vi "SerialServer.vi"(5 "Stop Refnum":refnum<vi>, 6 "Local Port":u16=16505, 7 "FPGA VI Reference In":refnum<k20>) -> (3 "FPGA VI Reference Out":refnum<k20>)   [LabVIEW 2012]
panel:
  out "error out":errorcluster
  out "OverRunError":bool
  in  "Flush on close":bool
  out "UART TX count":u64
  out "UART RX count":u64
  out "TCP Bytes Out":u64
  out "Elements in UART TX Queue":i32
  out "Elements in UART RX Queue":i32
  out "TCP Bytes In":u64
  out "connection ID":refnum<k5>
  out "Connected?":bool
  out "Stopped?":bool caption="BeenStopped?"
  out "remote address":string
  out "Remote Port":u16
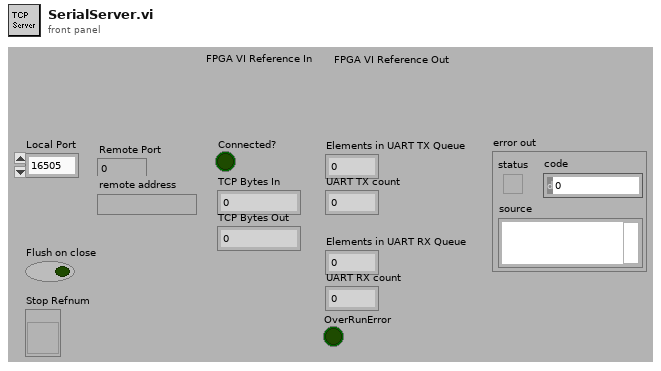
[diagram p1: front panel]
types:
  T1 = enum16{"Standard", "Buffered", "CRLF", "Immediate"}
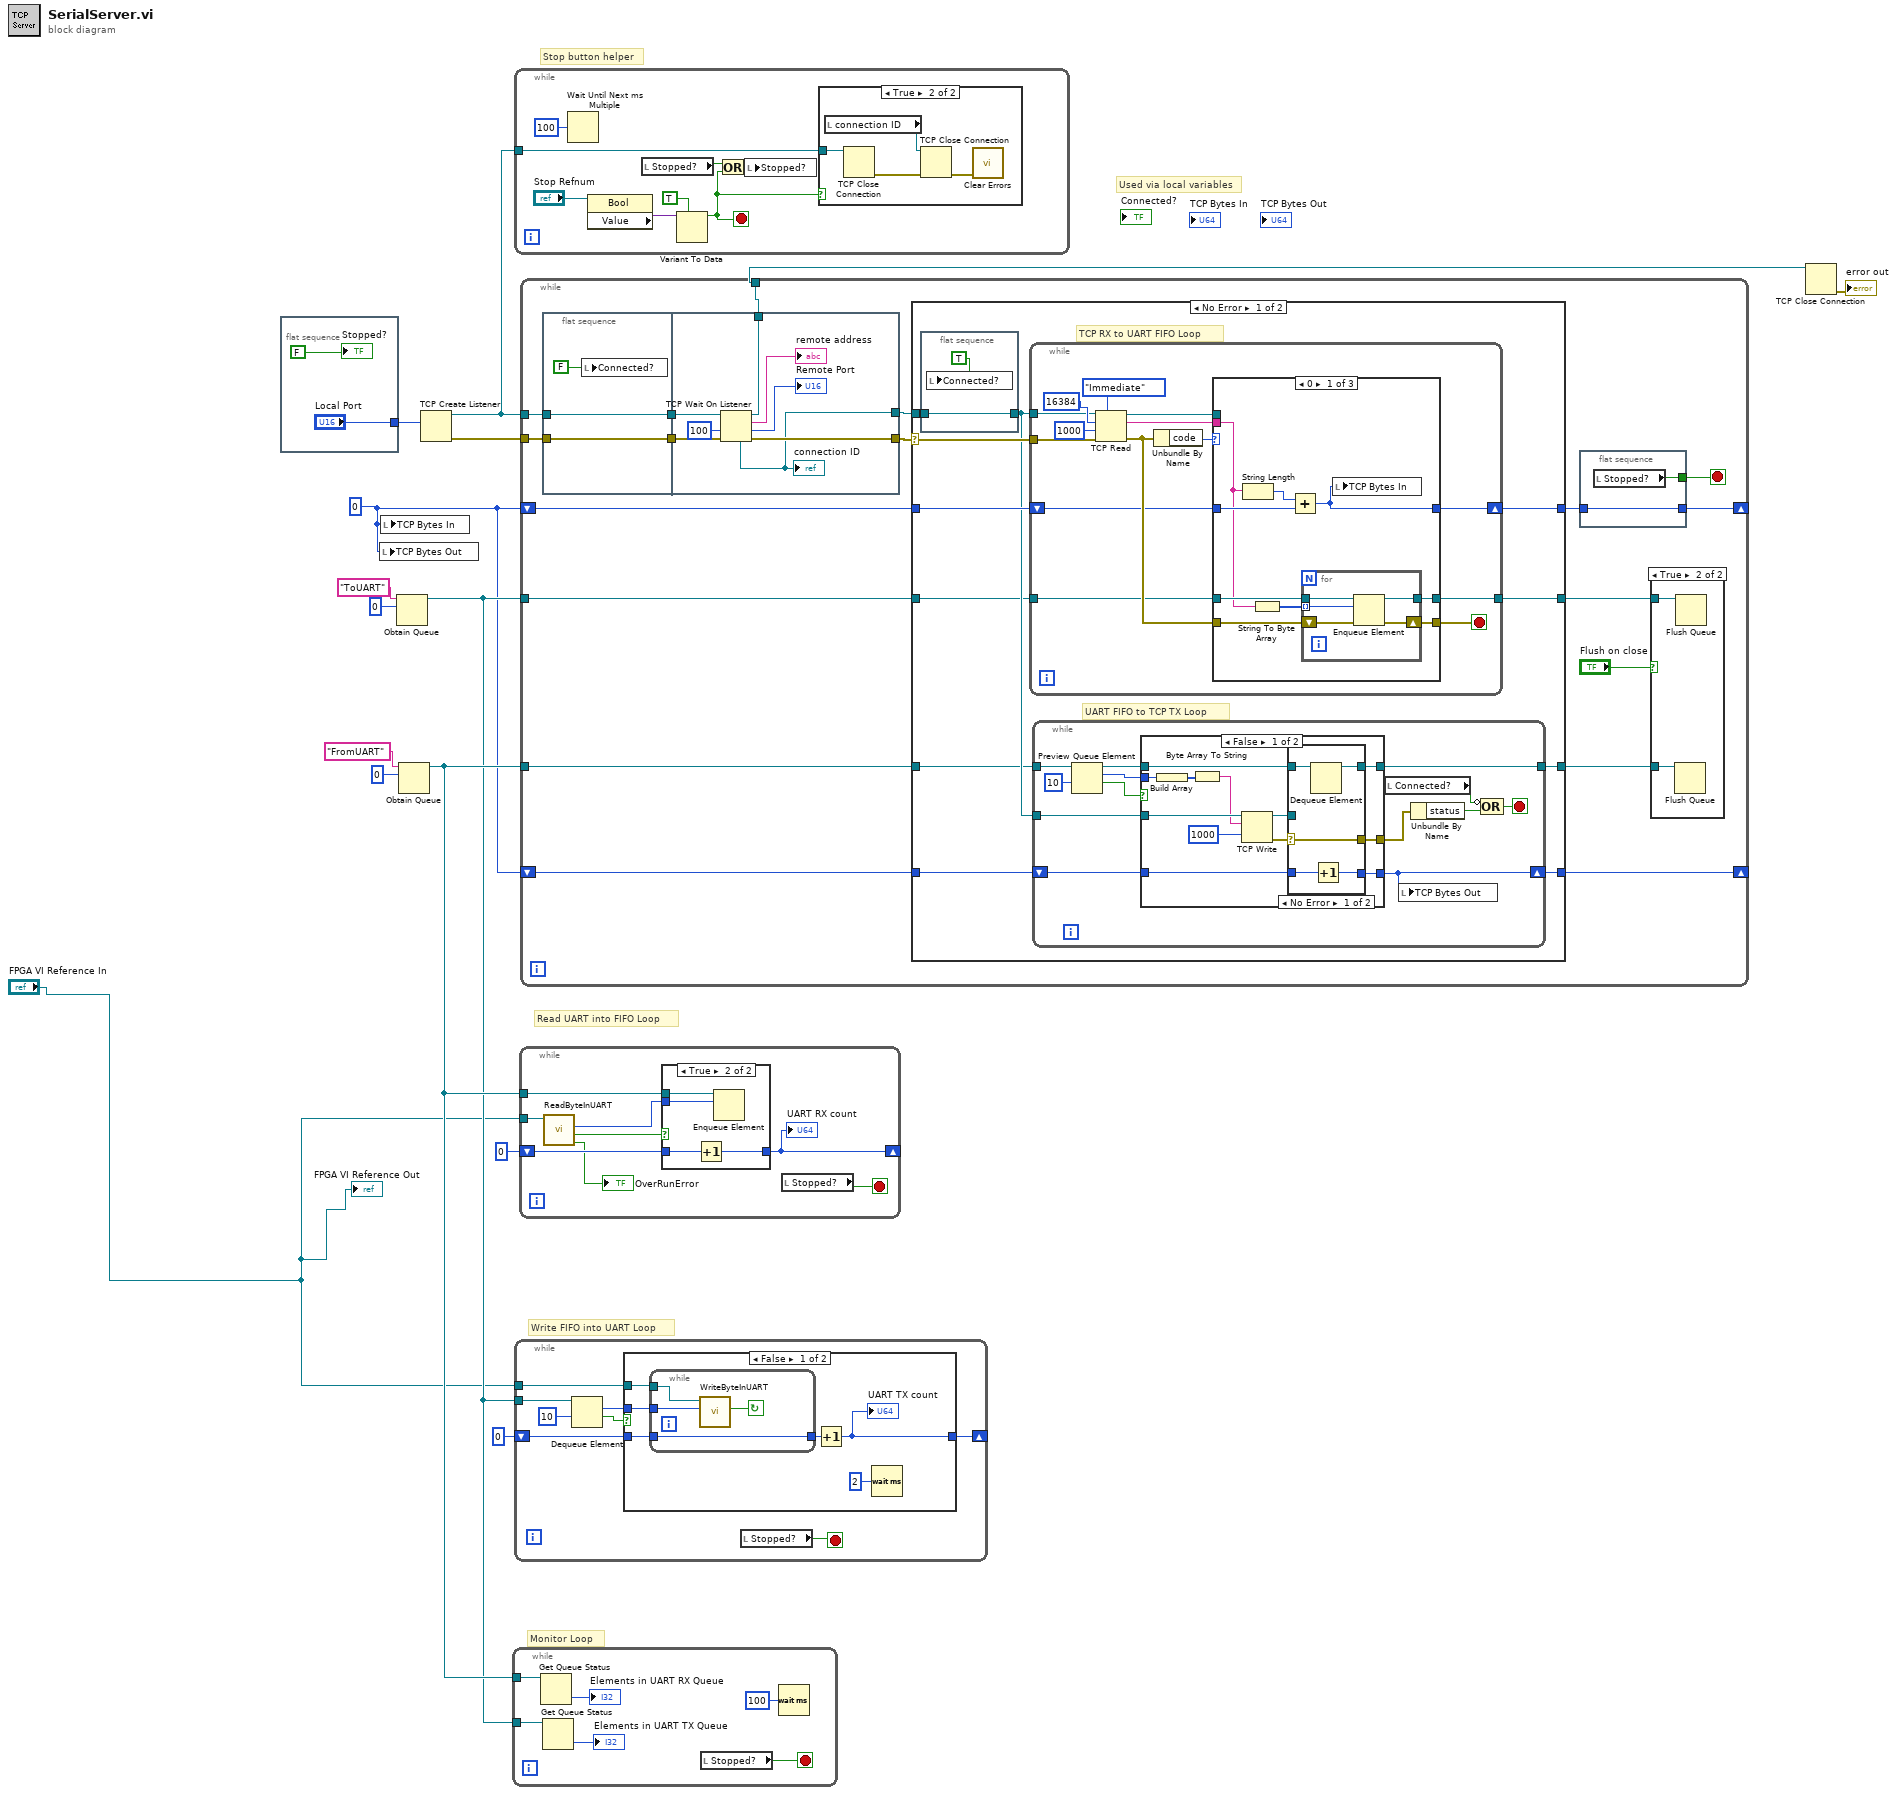
[diagram p0: block diagram]
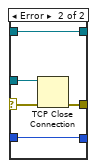
[diagram p6: hidden frame]
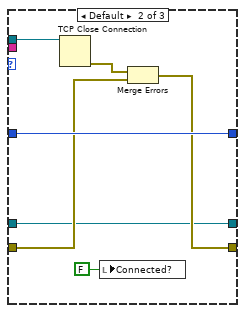
[diagram p8: hidden frame]
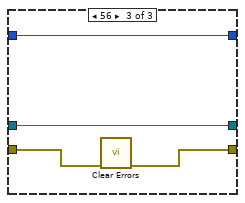
[diagram p9: hidden frame]
diagram:
  w7 = u64 0
  # "Monitor Loop"
  # "Write FIFO into UART Loop"
  # "Read UART into FIFO Loop"
  # "Stop button helper"
  # "Used via local variables"
  n1 = flat-sequence {
    tunnel: ["Local Port"] -> w2
    frame #0 {
      "Stopped?" <- FALSE ("Stopped?")
    }
  }
  n2 = local write "TCP Bytes Out"(w7) -> ()
  n3 = local write "TCP Bytes In"(w7) -> ()
  n4 = Obtain Queue(name (unnamed)="ToUART", element data type=u8 0) -> (queue out=w8:refnum<queue>)  [unwired: 3 in, 2 out]
  n5 = Obtain Queue(name (unnamed)="FromUART", element data type=u8 0) -> (queue out=w9:refnum<queue>)  [unwired: 3 in, 2 out]
  n6 = TCP Create Listener(10:w2) -> (0:w15:errorcluster, 3:w14:refnum<k5>)  [unwired: 1 in, 4 out]
  n7 = while {
    tunnel: w9 -> [w21]
    tunnel: w8 -> [w19]
    stop <- w23 stop-if-true
    n8 = Get Queue Status(queue=w21) -> (# elements in queue=→"Elements in UART RX Queue":i32)  [unwired: 1 in, 8 out]
    n9 = Get Queue Status(queue=w19) -> (# elements in queue=→"Elements in UART TX Queue":i32)  [unwired: 1 in, 8 out]
    n10 = local read "Stopped?"() -> (w23:bool)
    n11 = Wait (ms)(milliseconds to wait=u32 100) -> ()  [unwired: 1 out]
  }
  n12 = while {
    tunnel: w14 -> [w30]
    stop <- w24 stop-if-true
    n13 = Wait Until Next ms Multiple(millisecond multiple=u32 100) -> ()  [unwired: 1 out]
    n14 = property class="Bool"(reference="Stop Refnum") -> ("Value"=w29:variant)  [unwired: 1 in, 2 out]
    n15 = local read "Stopped?"() -> (w25:bool)
    n16 = Variant To Data(type=TRUE ("stop"), Variant=w29) -> (data=w24:bool)  [unwired: 1 in, 1 out]
    n17 = Or(x=w25, y=w24) -> (x .or. y?=w26:bool)
    n18 = local write "Stopped?"(w26) -> ()
    n19 = case shown="True" w24 {
      tunnel: w30 -> [_ w32]
      frame False {
      }
      frame True {
        n20 = local read "connection ID"() -> (w34:refnum<k5>)
        n21 = TCP Close Connection(connection ID=w32) -> (error out=w33:errorcluster)  [unwired: 1 in, 2 out]
        n22 = TCP Close Connection(connection ID=w34, error in (no error)=w33) -> (error out=w35:errorcluster)  [unwired: 2 out]
        n23 = call <vilib>:"Clear Errors.vi"("error in (no error)"=w35) -> ()  [unwired: 7 out]
      }
    }
  }
  n24 = while {
    tunnel: w8 -> [w43]
    shift-right: [w37] -> _
    shift-left: u64 0 -> [w38]
    tunnel: "FPGA VI Reference In" -> [w36]
    stop <- w39 stop-if-true
    n25 = Dequeue Element(queue=w43, timeout in ms (-1)=10) -> (element=w40:u8, timed out?=w41:bool)  [unwired: 1 in, 2 out]
    n26 = case shown="False" w41 {
      tunnel: w40 -> [w49 _]
      tunnel: w38 -> [w48 w54]
      tunnel: [w46 w54] -> w37
      tunnel: w36 -> [w44 _]
      frame False {
        n27 = while {
          tunnel: w49 -> [w52]
          tunnel: w48 -> [w53]
          tunnel: [w53] -> w47
          tunnel: w44 -> [w50]
          stop <- w51 continue-if-true
          n28 = call "WriteByteInUART.vi"("Byte Value"=w52, "FPGA VI Reference In"=w50) -> ("Overflow?"=w51:bool)  [unwired: 2 in, 6 out]
        }
        n29 = Increment(x=w47) -> (x+1=w46:u64)
        "UART TX count" <- w46
        n30 = Wait (ms)(milliseconds to wait=u32 2) -> ()  [unwired: 1 out]
      }
      frame True {
      }
    }
    n31 = local read "Stopped?"() -> (w39:bool)
  }
  n32 = while {
    tunnel: w9 -> [w61]
    shift-right: [w59] -> _
    shift-left: u64 0 -> [w60]
    tunnel: "FPGA VI Reference In" -> [w58]
    stop <- w62 stop-if-true
    n33 = call "ReadByteInUART.vi"("FPGA VI Reference In"=w58) -> ("OverRunError"=→"OverRunError":bool, "Did Read Byte"=w55:bool, "Byte Value"=w57:u8)  [unwired: 8 out]
    n34 = case shown="True" w55 {
      tunnel: w61 -> [_ w67]
      tunnel: w57 -> [_ w66]
      tunnel: [w63 w65] -> w59
      tunnel: w60 -> [w63 w64]
      frame False {
      }
      frame True {
        n35 = Increment(x=w64) -> (x+1=w65:u64)
        n36 = Enqueue Element(queue=w67, element=w66) -> ()  [unwired: 1 in, 4 out]
      }
    }
    "UART RX count" <- w59
    n37 = local read "Stopped?"() -> (w62:bool)
  }
  n38 = while {
    tunnel: w14 -> [w84]
    tunnel: w15 -> [w85]
    shift-right: [w78] -> _
    shift-left: w7 -> [w80]
    tunnel: w8 -> [w77]
    tunnel: w9 -> [w74]
    shift-right: [w72] -> _
    shift-left: w7 -> [w73]
    tunnel: [w68] -> w4
    stop <- w81 stop-if-true
    n39 = flat-sequence {
      tunnel: w84 -> [w89]
      tunnel: w85 -> [w90]
      tunnel: [w90] -> w76
      tunnel: [w89] -> w75
      tunnel: w76 -> [w96]
      tunnel: w75 -> [w95]
      tunnel: [w94] -> w83
      tunnel: [w91] -> w82
      tunnel: [w92] -> w68
      frame #0 {
        n40 = local write "Connected?"(FALSE ("Connected?")) -> ()
      }
      frame #1 {
        n41 = TCP Wait On Listener(8:w96, 9:100 ("timeout ms (wait forever: -1)"), 11:w95) -> (0:w94:errorcluster, 1:→"Remote Port":u16, 2:→"remote address":string, 3:w92:refnum<k5>, 4:w91:refnum<k5>)  [unwired: 1 in]
        "connection ID" <- w91
      }
    }
    n42 = case shown="No Error" w83 {
      selector: w83 -> [w109 _]
      tunnel: w82 -> [w108 _]
      tunnel: w80 -> [w111 w193]
      tunnel: [w110 w193] -> w79
      tunnel: w77 -> [w103 w190]
      tunnel: w74 -> [w104 w191]
      tunnel: w73 -> [w106 w192]
      tunnel: [w105 w192] -> w72
      tunnel: [w102 w190] -> w71
      tunnel: [w101 w191] -> w70
      frame No Error {
        # "UART FIFO to TCP TX Loop"
        # "TCP RX to UART FIFO Loop"
        n43 = flat-sequence {
          tunnel: w108 -> [w149]
          tunnel: [w149] -> w107
          frame #0 {
            n44 = local write "Connected?"(TRUE ("Connected?")) -> ()
          }
        }
        n45 = while {
          tunnel: w109 -> [w157]
          shift-right: [w154] -> w110
          shift-left: w111 -> [w155]
          tunnel: w103 -> [w153]
          tunnel: w107 -> [w152]
          tunnel: [w151] -> w102
          stop <- w158 stop-if-true
          n46 = TCP Read(connection ID=w152, bytes to read=16384, error in (no error)=w157, 7:T1."Immediate" ("mode (standard)"), 9:1000 ("timeout ms (25000)")) -> (connection ID out=w160:refnum<k5>, data out=w159:string, error out=w161:errorcluster)
          n47 = Unbundle By Name(w161) -> ("code"=w162:i32)
          n48 = case shown="0" w162 {
            tunnel: w161 -> [w167 w183 w189]
            tunnel: w160 -> [_ w184 _]
            tunnel: w159 -> [w169 _ _]
            tunnel: [w166 w181 w188] -> w158
            tunnel: w155 -> [w173 w185 w187]
            tunnel: [w172 w185 w187] -> w154
            tunnel: w153 -> [w171 w179 w186]
            tunnel: [w165 w179 w186] -> w151
            frame 0 {
              n49 = String Length(string=w169) -> (length=w170:i32)
              n50 = String To Byte Array(string=w169) -> (unsigned byte array=w168:u8[])
              n51 = Add(x=w170, y=w173) -> (x+y=w172:u64)
              n52 = for {
                tunnel: w171 -> [w178]
                tunnel: w168 -> [w177] mode=indexing
                shift-right: [w175] -> w166
                shift-left: w167 -> [w176]
                tunnel: [w174] -> w165
                n53 = Enqueue Element(queue=w178, element=w177, error in (no error)=w176) -> (queue out=w174:refnum<queue>, error out=w175:errorcluster)  [unwired: 2 out]
              }
              n54 = local write "TCP Bytes In"(w172) -> ()
            }
            frame Default {
              n55 = TCP Close Connection(connection ID=w184) -> (error out=w182:errorcluster)  [unwired: 1 in, 2 out]
              n56 = local write "Connected?"(FALSE ("Connected?")) -> ()
              n57 = Merge Errors(w182, w183) -> (w181:errorcluster)
            }
            frame 56 {
              n58 = call <vilib>:"Clear Errors.vi"("error in (no error)"=w189) -> ("error out"=w188:errorcluster)  [unwired: 6 out]
            }
          }
        }
        n59 = while {
          tunnel: w107 -> [w120]
          tunnel: w104 -> [w123]
          tunnel: [w112] -> w101
          shift-right: [w116] -> w105
          shift-left: w106 -> [w118]
          stop <- w113 stop-if-true
          n60 = Preview Queue Element(queue=w123, timeout in ms (-1)=10) -> (queue out=w117:refnum<queue>, element=w121:u8, timed out?=w122:bool)  [unwired: 1 in, 1 out]
          n61 = case shown="False" w122 {
            tunnel: w121 -> [w135 _]
            tunnel: w120 -> [w136 _]
            tunnel: [w130 _] -> w119
            tunnel: w118 -> [w127 w148]
            tunnel: [w126 w148] -> w116
            tunnel: w117 -> [w128 w147]
            tunnel: [w125 w147] -> w112
            frame False {
              n62 = Build Array(w135) -> (w134:u8[])
              n63 = Byte Array To String(unsigned byte array=w134) -> (string=w133:string)
              n64 = TCP Write(connection ID=w136, data in=w133, 9:1000 ("timeout ms (25000)")) -> (connection ID out=w129:refnum<k5>, error out=w131:errorcluster)  [unwired: 1 in, 1 out]
              n65 = case shown="No Error" w131 {
                selector: w131 -> [w141 w145]
                tunnel: [w141 w144] -> w130
                tunnel: w129 -> [_ w146]
                tunnel: w128 -> [w140 w142]
                tunnel: w127 -> [w139 w143]
                tunnel: [w138 w143] -> w126
                tunnel: [w137 w142] -> w125
                frame No Error {
                  n66 = Dequeue Element(queue=w140) -> (queue out=w137:refnum<queue>)  [unwired: 2 in, 3 out]
                  n67 = Increment(x=w139) -> (x+1=w138:u64)
                }
                frame Error {
                  n68 = TCP Close Connection(connection ID=w146, error in (no error)=w145) -> (error out=w144:errorcluster)  [unwired: 2 out]
                }
              }
            }
            frame True {
            }
          }
          n69 = local read "Connected?"() -> (w115:bool)
          n70 = local write "TCP Bytes Out"(w116) -> ()
          n71 = Unbundle By Name(w119) -> ("status"=w114:bool)
          n72 = Compound Arithmetic op=OR(invert w115, w114) -> (w113:bool)
        }
      }
      frame Error {
      }
    }
    n73 = flat-sequence {
      tunnel: [w100] -> w81
      tunnel: w79 -> [w99]
      tunnel: [w99] -> w78
      frame #0 {
        n74 = local read "Stopped?"() -> (w100:bool)
      }
    }
    n75 = case shown="True" "Flush on close" {
      tunnel: w71 -> [_ w87]
      tunnel: w70 -> [_ w86]
      frame False {
      }
      frame True {
        n76 = Flush Queue(queue=w86) -> ()  [unwired: 1 in, 3 out]
        n77 = Flush Queue(queue=w87) -> ()  [unwired: 1 in, 3 out]
      }
    }
  }
  n78 = TCP Close Connection(connection ID=w4) -> (error out=→"error out":errorcluster)  [unwired: 2 in, 1 out]
  "FPGA VI Reference Out" <- "FPGA VI Reference In"
